vi "Host.vi"() -> ()   [LabVIEW 2025]
uses:
  <vilib>/FPGAPlugInAG/cRIO-9035/niLvFpga_Open_cRIO-9035.vi
  <vilib>/rvi/interface/common/dynamic/niFpgaDynamicAddResources.vi
  <vilib>/FPGAPlugInAG/Dynamic/niLvFpga_Reset_Dynamic.vi
  <vilib>/Utility/error.llb/Error Cluster From Error Code.vi
  <vilib>/rvi/errors/niLvFpgaAdjustHostInterfaceError.vi
  <vilib>/FPGAPlugInAG/Dynamic/niLvFpga_Run_Dynamic.vi
  <vilib>/FPGAPlugInAG/Dynamic/niLvFpga_Close_Dynamic.vi
  <vilib>/rvi/interface/nirviOpenFPGA/nirviOpenFPGA.xnode
  FPGA Bitfiles/hmmlponfpgav4_FPGATarget_Target_XqGQJ98FoTY.lvbitx
  Target.vi
  <vilib>/rvi/interface/nirviMethod/nirviMethod.xnode
  <vilib>/rvi/interface/nirviCloseFPGA/nirviCloseFPGA.xnode
  <vilib>/rvi/errors/niLvFpgaMergeErrorWithErrorCode.vi
  <vilib>/FPGAPlugInAG/Dynamic/niLvFpga_ReadFifo_Dynamic.vi
  <vilib>/FPGAPlugInAG/Dynamic/niLvFpga_WriteFifo_Dynamic.vi
panel:
  out "Data":u32[](array[numeric])
  out "Window(s)":dbl[][](array[numeric])
  out "input":dbl[][](array[numeric])
  out "Healthy%":sgl[](array[numeric])
  out "Window":dbl[](graph)
  out "size(s) 2":i32
  out "output array":sgl[](array[numeric])
  out "Unhealthy%":sgl[](array[numeric])
  out "size(s)":i32[](array[numeric])
  out "Uncontrolled Acceleration":dynamicdata(graph)
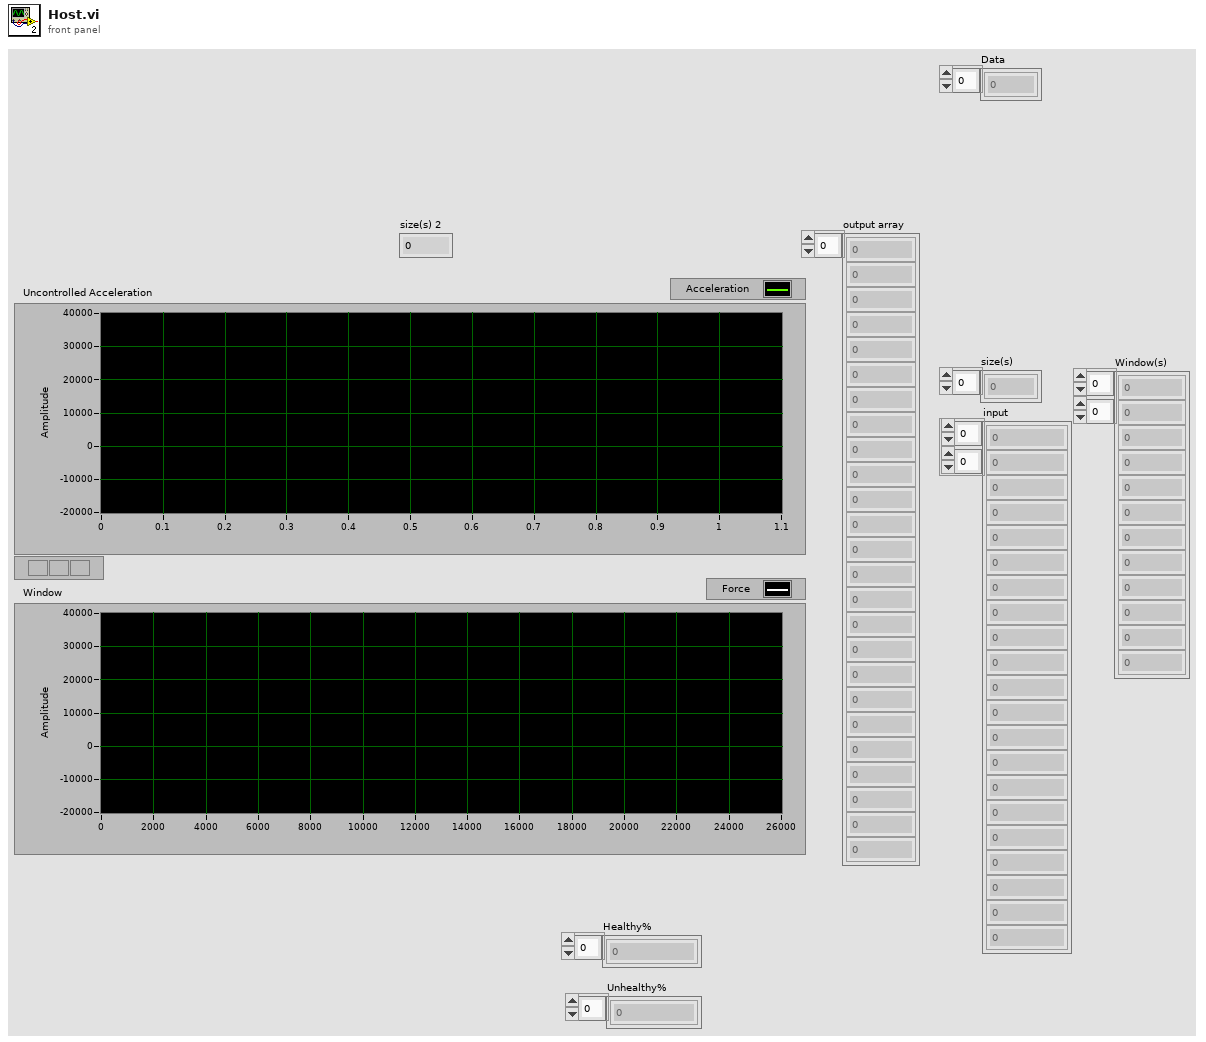
[diagram p1: front panel]
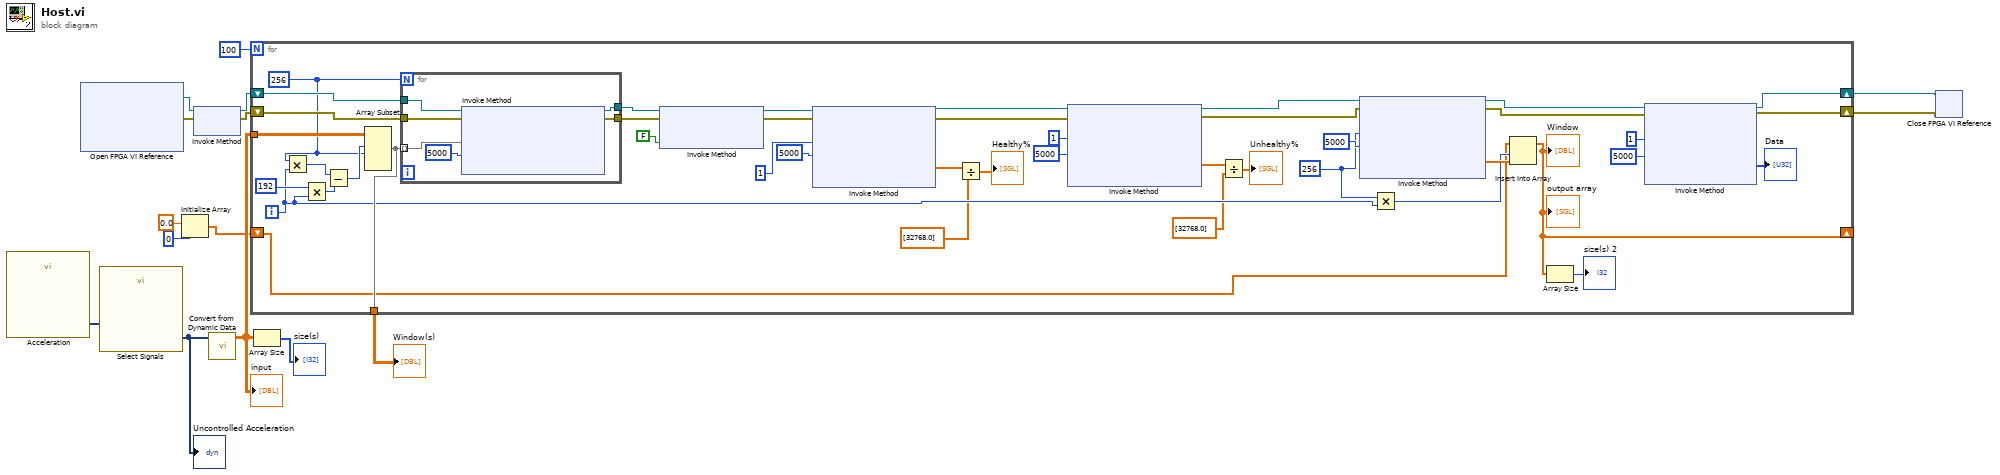
[diagram p0: block diagram]
diagram:
  n1 = call "Acceleration"() -> ("Signals"=w15:dynamicdata)  [unwired: 6 in, 5 out]
  n2 = xnode "Open FPGA VI Reference"() -> ("FPGA VI Reference Out"=w14:refnum<k20>, "error out"=w11:errorcluster)  [unwired: 2 in]
  n3 = call "Select Signals"("Signals"=w15) -> ("Signal Out"=w10:dynamicdata)  [unwired: 9 in, 1 out]
  "Uncontrolled Acceleration" <- w10
  n4 = Initialize Array(0.0 ("element"), 0 ("dimension size")) -> (w3:dbl[])
  n5 = xnode "Invoke Method"("FPGA VI Reference In"=w14, "error in"=w11) -> ("FPGA VI Reference Out"=w13:refnum<k20>, "error out"=w12:errorcluster)
  n6 = call "Convert from Dynamic Data"("Dynamic Data Type"=w10) -> ("Array"=w5:dbl[][])  [unwired: 3 in]
  "input" <- w5
  n7 = for {
    N: 100 -> [_]
    shift-right: [w19] -> w8
    shift-left: w13 -> [w58]
    shift-right: [w18] -> w7
    shift-left: w12 -> [w57]
    tunnel: w5 -> [w49]
    tunnel: [w48] -> w4
    shift-right: [w42] -> _
    shift-left: w3 -> [w39]
    i -> [w37]
    w40 = u32 256 ("Number of Elements")
    w35 = 256
    n8 = Multiply(x=w35, y=w37) -> (x*y=w47:i32)
    n9 = Multiply(x=192 ("y"), y=w37) -> (x*y=w36:i32)
    n10 = Subtract(x=w47, y=w36) -> (x-y=w46:i32)
    n11 = Array Subset(array=w49, index (row)=w46, length (row)=w35) -> (w48:dbl[][])  [unwired: 2 in]
    n12 = for {
      N: w35 -> [_]
      tunnel: w58 -> [w64]
      tunnel: w57 -> [w63]
      tunnel: [w61] -> w53
      tunnel: [w60] -> w52
      tunnel: w48 -> [w59] mode=indexing
      n13 = xnode "Invoke Method"("FPGA VI Reference In"=w64, "error in"=w63, "Data"=w59, "Timeout (ms)"=5000) -> ("FPGA VI Reference Out"=w61:refnum<k20>, "error out"=w60:errorcluster)  [unwired: 1 out]
    }
    n14 = xnode "Invoke Method"("FPGA VI Reference In"=w53, "error in"=w52, "Wait Until Done (F)"=FALSE) -> ("FPGA VI Reference Out"=w55:refnum<k20>, "error out"=w54:errorcluster)
    n15 = xnode "Invoke Method"("FPGA VI Reference In"=w55, "error in"=w54, "Number of Elements"=u32 1, "Timeout (ms)"=5000) -> ("FPGA VI Reference Out"=w34:refnum<k20>, "error out"=w33:errorcluster, "Data"=w27:sgl[])  [unwired: 1 out]
    n16 = Divide(x=w27, y=sgl[] [32768.0]) -> (x/y=→"Healthy%":sgl[])
    n17 = xnode "Invoke Method"("FPGA VI Reference In"=w34, "error in"=w33, "Number of Elements"=u32 1, "Timeout (ms)"=5000) -> ("FPGA VI Reference Out"=w31:refnum<k20>, "error out"=w32:errorcluster, "Data"=w24:sgl[])  [unwired: 1 out]
    n18 = Divide(x=w24, y=sgl[] [32768.0]) -> (x/y=→"Unhealthy%":sgl[])
    n19 = xnode "Invoke Method"("FPGA VI Reference In"=w31, "error in"=w32, "Number of Elements"=w40, "Timeout (ms)"=5000) -> ("FPGA VI Reference Out"=w17:refnum<k20>, "error out"=w16:errorcluster, "Data"=w44:sgl[])  [unwired: 1 out]
    n20 = Multiply(x=w40, y=w37) -> (x*y=w43:u32)
    n21 = Insert Into Array(array=w39, index=w43, new element=w44) -> (w42:dbl[])
    "Window" <- w42
    "output array" <- w42
    n22 = Array Size(array=w42) -> (size(s)=→"size(s) 2":i32)
    n23 = xnode "Invoke Method"("FPGA VI Reference In"=w17, "error in"=w16, "Number of Elements"=u32 1, "Timeout (ms)"=5000) -> ("FPGA VI Reference Out"=w19:refnum<k20>, "error out"=w18:errorcluster, "Data"=→"Data":u32[])  [unwired: 1 out]
  }
  "Window(s)" <- w4
  n24 = Array Size(array=w5) -> (size(s)=→"size(s)":i32[])
  n25 = xnode "Close FPGA VI Reference"("FPGA VI Reference In"=w8, "error in"=w7) -> ()  [unwired: 1 out]
